vi "GRNF_DI.vi"(7 "RefNum Name":string) -> (0 "Error":errorcluster, 3 "Device Reference":T1={"DevStatus"={"status"=FALSE, "code"=0, "source"=""}, "DIO Channel"=enum."Invalid", "CntIndex"=enum."Invalid", "Normally Closed"=FALSE})   [LabVIEW 2019]
uses:
  <vilib>/Rock Robotics/WPI/Switch/WPI_SwitchDevRef.ctl
  <vilib>/Rock Robotics/SystemInterfaces/DIO/FPGA_DIOChannel.ctl
  <vilib>/Rock Robotics/SystemInterfaces/Counter/FPGA_CounterCtrSystemIndex.ctl
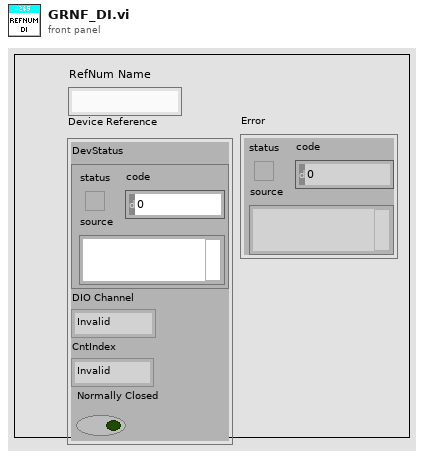
[diagram p1: front panel]
types:
  T1 = typedef "WPI_SwitchDevRef.ctl" = cluster{"DevStatus":errorcluster, "DIO Channel":T2, "CntIndex":T3, "Normally Closed":bool}
  T2 = typedef "FPGA_DIOChannel.ctl" = enum8{"DIO 0", "DIO 1", "DIO 2", "DIO 3", "DIO 4", "DIO 5", "DIO 6", "DIO 7", "DIO 8", "DIO 9", "DIO MXP 0", "DIO MXP 1", "DIO MXP 2", "DIO MXP 3", "DIO MXP 4", "DIO MXP 5", "DIO MXP 6", "DIO MXP 7", "DIO MXP 8", "DIO MXP 9", "DIO MXP 10", "DIO MXP 11", "DIO MXP 12", "DIO MXP 13", "DIO MXP 14", "DIO MXP 15", "SPI Port CS1", "SPI Port CS2", "SPI Port CS3", "SPI Port MISO", "SPI Port MOSI", "Invalid"}
  T3 = typedef "FPGA_CounterCtrSystemIndex.ctl" = enum8{"Ctr 0", "Ctr 1", "Ctr 2", "Ctr 3", "Ctr 4", "Ctr 5", "Ctr 6", "Ctr 7", "Invalid"}
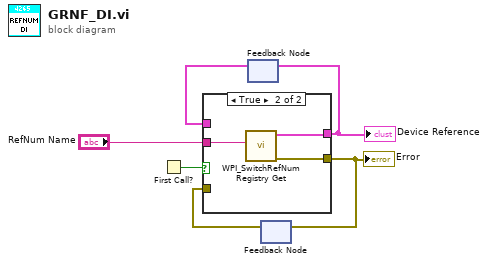
[diagram p0: block diagram]
diagram:
  n1 = First Call?() -> (First Call?: T/F=w6:bool)
  n2 = feedback #1() -> (w5:T1)  [unwired: 1 in]
  n3 = feedback #2() -> (w2:errorcluster)  [unwired: 1 in]
  n4 = case shown="True" w6 {
    tunnel: [w8 w11] -> w1
    tunnel: w5 -> [w8 _]
    tunnel: "RefNum Name" -> [_ w9]
    tunnel: [w7 w10] -> w3
    tunnel: w2 -> [w7 _]
    frame False {
    }
    frame True {
      n5 = call <vilib>:"WPI_SwitchRefNum Registry Get.vi"("refnum name"=w9) -> ("error out"=w10:errorcluster, "SwitchDevRef"=w11:T1)  [unwired: 9 in]
    }
  }
  "Error" <- w3
  "Device Reference" <- w1
  n6 = feedback-in #1(w1) -> ()
  n7 = feedback-in #2(w3) -> ()
